vi "LEP_RV_MemoryMap_GetAvailable.vi"(11 "error in (no error)":errorcluster) -> (4 "Code Section List":i32[](array[numeric]), 6 "Data Section List":i32[](array[numeric]), 8 "Section Names":string[](array[string]), 13 "Default Code Section":i32, 14 "Default Data Section":i32, 15 "error out":errorcluster)   [LabVIEW 2011]
doc: "Define default memory mapping for the Axiom CMD565 target."
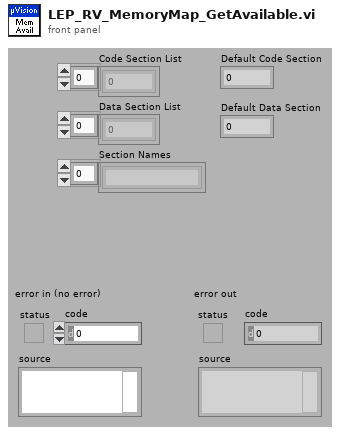
[diagram p1: front panel]
types:
  T1 = enum16{"Normal", "Minimized", "Maximized", "Hidden", "Locked"}
  T2 = cluster{"Start Address":u64, "Size":u64, "Type":enum16{"UV_MR_NONE", "UV_MR_ROM", "UV_MR_RAM"}, "Default RAM":bool, "Default ROM":bool, "Is ZI RAM":bool}[]
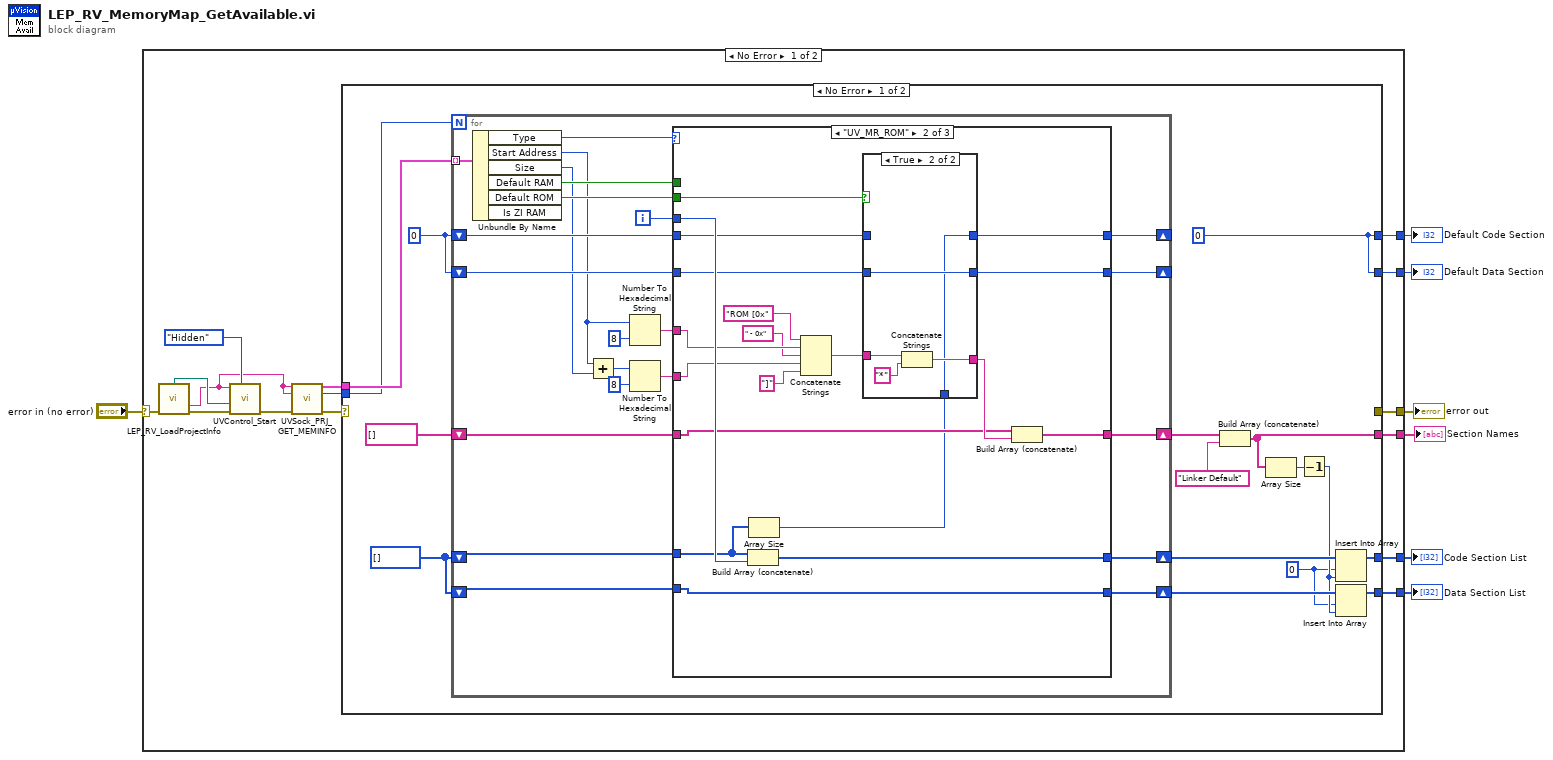
[diagram p0: block diagram]
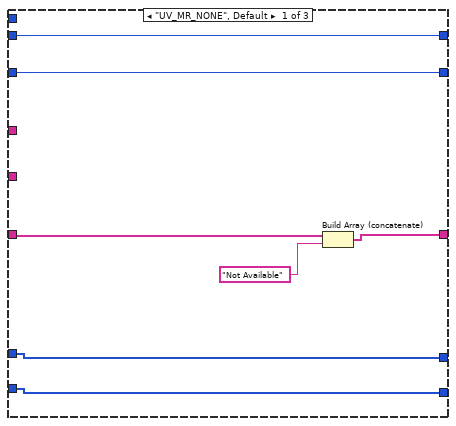
[diagram p2: hidden frame]
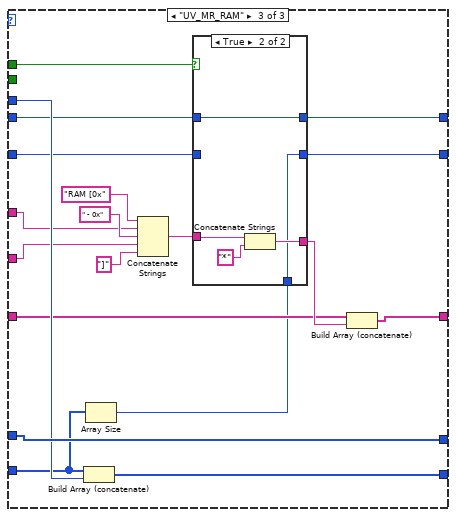
[diagram p4: hidden frame]
diagram:
  n1 = case shown="No Error" "error in (no error)" {
    selector: "error in (no error)" -> [w12 w123]
    tunnel: [w20 _] -> w7
    tunnel: [w19 _] -> w6
    tunnel: [w18 _] -> w5
    tunnel: [w17 _] -> w4
    tunnel: [w15 w123] -> w2
    tunnel: [w14 _] -> w1
    frame No Error {
      n2 = call "LEP_RV_LoadProjectInfo.vi"("error in (no error)"=w12) -> ("Project File"=w10:path, "Target Name"=w8:string, "error out"=w13:errorcluster)  [unwired: 8 in, 4 out]
      n3 = call "UVControl_Start.vi"("Mode"=T1."Hidden", "error in (no error)"=w13, "Project File"=w10, "Target"=w8) -> ("error out"=w11:errorcluster)  [unwired: 5 in, 2 out]
      n4 = call "UVSock_PRJ_GET_MEMINFO.vi"("Target"=w8, "Target Name"=w8, "error in (no error)"=w11) -> ("Memory Ranges"=w22:T2, "Memory Range Count"=w21:u32, "error out"=w16:errorcluster)  [unwired: 10 in]
      n5 = case shown="No Error" w16 {
        selector: w16 -> [_ w122]
        tunnel: w22 -> [w38 _]
        tunnel: w21 -> [w37 _]
        tunnel: [w24 _] -> w20
        tunnel: [w24 _] -> w19
        tunnel: [w28 _] -> w18
        tunnel: [w26 _] -> w17
        tunnel: [_ w122] -> w15
        tunnel: [w30 _] -> w14
        frame No Error {
          w34 = i32[] []
          w23 = 0 ("index")
          w24 = 0
          w33 = 0
          n6 = for {
            N: w37 -> [_]
            tunnel: w38 -> [w60] mode=indexing
            shift-right: [w58] -> w29
            shift-left: w34 -> [w57]
            shift-right: [w55] -> w36
            shift-left: w34 -> [w54]
            shift-right: [w51] -> _
            shift-left: w33 -> [w50]
            shift-right: [w49] -> _
            shift-left: w33 -> [w48]
            shift-right: [w40] -> w32
            shift-left: string[] [] -> [w39]
            i -> [w56]
            n7 = Unbundle By Name(w60) -> ("Type"=w59:enum16{"UV_MR_NONE", "UV_MR_ROM", "UV_MR_RAM"}, "Start Address"=w44:u64, "Size"=w43:u64, "Default RAM"=w53:bool, "Default ROM"=w52:bool)  [unwired: 1 out]
            n8 = Add(x=w44, y=w43) -> (x+y=w47:u64)
            n9 = Number To Hexadecimal String(1:i16 8 ("width (-)"), 2:w44) -> (0:w42:string)
            n10 = Number To Hexadecimal String(1:i16 8 ("width (-)"), 2:w47) -> (0:w41:string)
            n11 = case shown="\"UV_MR_ROM\"" w59 {
              tunnel: [w67 w86 w112] -> w58
              tunnel: w57 -> [w67 w69 w112]
              tunnel: w56 -> [_ w83 w111]
              tunnel: [w66 w85 w113] -> w55
              tunnel: w54 -> [w66 w85 w96]
              tunnel: w53 -> [_ _ w110]
              tunnel: w52 -> [_ w84 _]
              tunnel: [w65 w82 w108] -> w51
              tunnel: w50 -> [w65 w81 w107]
              tunnel: [w64 w80 w109] -> w49
              tunnel: w48 -> [w64 w79 w106]
              tunnel: w42 -> [_ w77 w102]
              tunnel: w41 -> [_ w75 w101]
              tunnel: [w63 w71 w97] -> w40
              tunnel: w39 -> [w62 w70 w98]
              frame "UV_MR_NONE", Default {
                n12 = Build Array (concatenate)(w62, "Not Available") -> (w63:string[])
              }
              frame "UV_MR_ROM" {
                n13 = Build Array (concatenate)(w69, w83) -> (w86:i32[])
                n14 = Array Size(array=w69) -> (size(s)=w68:i32)
                n15 = Concatenate Strings("ROM [0x" ("string"), w77, " - 0x" ("string"), w75, "]" ("string")) -> (w73:string)
                n16 = case shown="True" w84 {
                  tunnel: [w89 w90] -> w82
                  tunnel: w81 -> [w89 _]
                  tunnel: [w88 w94] -> w80
                  tunnel: w79 -> [w88 w94]
                  tunnel: w73 -> [w87 w93]
                  tunnel: [w87 w91] -> w72
                  tunnel: w68 -> [_ w90]
                  frame False {
                  }
                  frame True {
                    n17 = Concatenate Strings(w93, "*" ("string")) -> (w91:string)
                  }
                }
                n18 = Build Array (concatenate)(w70, w72) -> (w71:string[])
              }
              frame "UV_MR_RAM" {
                n19 = Build Array (concatenate)(w96, w111) -> (w113:i32[])
                n20 = Array Size(array=w96) -> (size(s)=w95:i32)
                n21 = Concatenate Strings("RAM [0x" ("string"), w102, " - 0x" ("string"), w101, "]" ("string")) -> (w100:string)
                n22 = case shown="True" w110 {
                  tunnel: [w115 w117] -> w109
                  tunnel: [w116 w121] -> w108
                  tunnel: w107 -> [w116 w121]
                  tunnel: w106 -> [w115 _]
                  tunnel: w100 -> [w114 w119]
                  tunnel: [w114 w118] -> w99
                  tunnel: w95 -> [_ w117]
                  frame False {
                  }
                  frame True {
                    n23 = Concatenate Strings(w119, "*" ("string")) -> (w118:string)
                  }
                }
                n24 = Build Array (concatenate)(w98, w99) -> (w97:string[])
              }
            }
          }
          n25 = Build Array (concatenate)(w32, "Linker Default") -> (w30:string[])
          n26 = Array Size(array=w30) -> (size(s)=w27:i32)
          n27 = Decrement(x=w27) -> (x-1=w25:i32)
          n28 = Insert Into Array(array=w29, index=w23, new element=w25) -> (w28:i32[])
          n29 = Insert Into Array(array=w36, index=w23, new element=w25) -> (w26:i32[])
        }
        frame Error {
        }
      }
    }
    frame Error {
    }
  }
  "error out" <- w2
  "Code Section List" <- w5
  "Data Section List" <- w4
  "Default Code Section" <- w7
  "Default Data Section" <- w6
  "Section Names" <- w1
